vi "ReadConfig.vi"(8 "error in (no error)":errorcluster, 11 "SiemensDigitalEnergyMeter in":refnum<class "SiemensDigitalEnergyMeter.lvclass">) -> (0 "error out":errorcluster, 2 "Config":variant, 3 "SiemensDigitalEnergyMeter out":refnum<class "SiemensDigitalEnergyMeter.lvclass">)   [LabVIEW 2018, in "SensorPlugins.lvlib" / "SiemensDigitalEnergyMeter.lvclass"]
doc: "This VI reads the class cluster from the Siemens Digital Energy Meter."
uses:
  SiemensDigitalEnergyMeter.lvclass
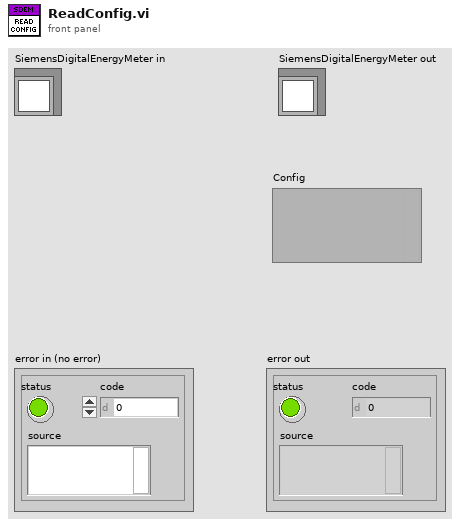
[diagram p1: front panel]
types:
  T1 = typedef "SensorPlugins.lvlib/SiemensDigitalEnergyMeter.lvclass/SiemensDigitalEnergyMeterControls.ctl" = cluster{"Measurement(s)":u16[], "Configuration Commands":string, "Use Measurement Commands Text Box?":bool, "Measurement Commands":string, "Connected?":bool, "Serial Number":string, "IP Address":string, "Port (502)":u16, "Unit ID":u8, "Serial Type":enum16{"RTU", "ASCII"}, "VISA Resource Name":refnum<visa-resource-name>, "Using TCP?":bool}[]
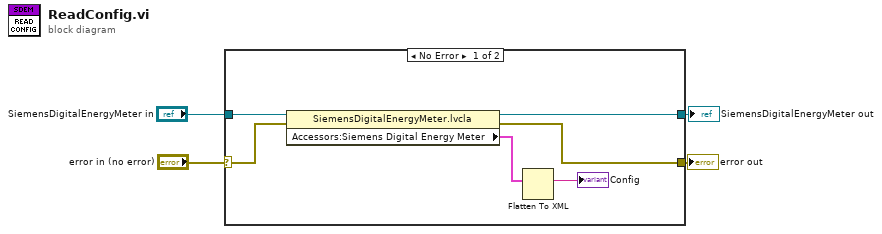
[diagram p0: block diagram]
diagram:
  n1 = case shown="No Error" "error in (no error)" {
    selector: "error in (no error)" -> [w8 w12]
    tunnel: "SiemensDigitalEnergyMeter in" -> [w10 w11]
    tunnel: [w7 w12] -> w2
    tunnel: [w9 w11] -> w1
    frame No Error {
      n2 = property class="SiemensDigitalEnergyMeter.lvcla"(reference=w10, error in=w8) -> (reference out=w9:refnum<class "SiemensDigitalEnergyMeter.lvclass">, error out=w7:errorcluster, "Accessors:Siemens Digital Energy Meter"=w6:T1)
      n3 = Flatten To XML(anything=w6) -> (xml string=→"Config":string)
    }
    frame Error {
    }
  }
  "error out" <- w2
  "SiemensDigitalEnergyMeter out" <- w1
